vi "Get SCC Revision number.vi"(10 "path":path) -> (2 "Revision":i32)   [LabVIEW 2013]
panel:
  in  "LibSubWCRev.ISubWCRev":refnum<k7>
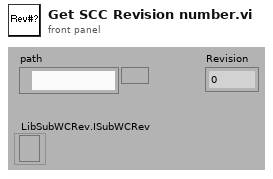
[diagram p1: front panel]
types:
  T1 = enum32{"invalid app kind", "Development System", "Run Time System", "Student Edition", "Embedded LabVIEW", "Evaluation", "Custom"}
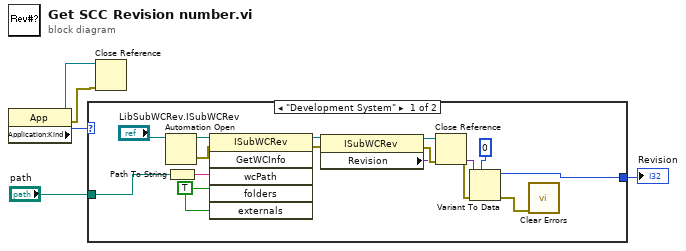
[diagram p0: block diagram]
diagram:
  n1 = property class="App"() -> (reference out=w1:refnum<vi>, error out=w2:errorcluster, "Application:Kind"=w4:T1)  [unwired: 2 in]
  n2 = case shown="\"Development System\"" w4 {
    tunnel: [w10 _] -> w5
    tunnel: "path" -> [w6 _]
    frame "Development System" {
      w11 = TRUE ("folders")
      n3 = Automation Open(Automation Refnum="LibSubWCRev.ISubWCRev") -> (Automation Refnum=w16:refnum<k7>, error out=w18:errorcluster)  [unwired: 3 in]
      n4 = Path To String(path=w6) -> (string=w20:string)
      n5 = invoke class="ISubWCRev" method="GetWCInfo"(reference=w16, error in=w18, "wcPath"=w20, "folders"=w11, "externals"=w11) -> (reference out=w17:refnum<k7>, error out=w19:errorcluster)  [unwired: 1 in, 4 out]
      n6 = property class="ISubWCRev"(reference=w17, error in=w19) -> (reference out=w14:refnum<k7>, error out=w15:errorcluster, "Revision"=w7:variant)
      n7 = Close Reference(reference=w14, error in (no error)=w15) -> (error out=w12:errorcluster)
      n8 = Variant To Data(error in=w12, type=0, Variant=w7) -> (data=w10:i32, error out=w8:errorcluster)
      n9 = call <vilib>:"Clear Errors.vi"("error in (no error)"=w8) -> ()  [unwired: 6 in, 1 out]
    }
    frame "Run Time System", Default {
    }
  }
  "Revision" <- w5
  n10 = Close Reference(reference=w1, error in (no error)=w2) -> ()  [unwired: 1 out]
